vi "Add cell to tableV2.vi"(0 "PdfP Table":refnum<k24>, 1 "Row format with ref":T8, 2 "Image to Add [ ]":T9, 3 "Back Ground Color":u32(colorbox)=16777215, 5 "String [ ]":string[](array[string]), 7 "i":i32, 9 "Column Width (points)":dbl, 11 "error in (no error)":errorcluster, 13 "PDF Report IN":refnum<class "PDF Report Class.lvclass">) -> (4 "PdfP Table duplicate":refnum<k24>, 15 "error out":errorcluster)   [LabVIEW 2019]
doc: "Version 1.0\nDeveloped by Jean-Marc Simard\nCopyright © 2010, Exaprom Inc.\nAll rights reserved.\nLicense: BSD\n\nWith iTextSharp 4.1.6 (http://itextsharp.sourceforge.net)\nunder Mozilla Public License Version 1.1\n(http://www.mozilla.org/MPL/MPL-1.1.html)"
uses:
  C:/work/niobrara_lv/labview pdf writer fixing/DLL/itextsharp.dll
  DLL/itextsharp.dll
  Controls/Font Controls/Font size.ctl
  Controls/Table Controls/Cell Vertical alignment.ctl
  Controls/Text Controls/Texte alignement.ctl
  Controls/General Controls/Image to Add refnum [ ].ctl
  Controls/Table Controls/Table Custom type Titles or Datas.ctl
  Controls/Text Controls/Unicode/Character type.ctl
  Controls/Text Controls/Unicode/Writing direction.ctl
  Controls/Text Controls/Unicode/ASCII or Unicode.ctl
  LV Class/PDF Report Class/PDF Report Class.lvclass
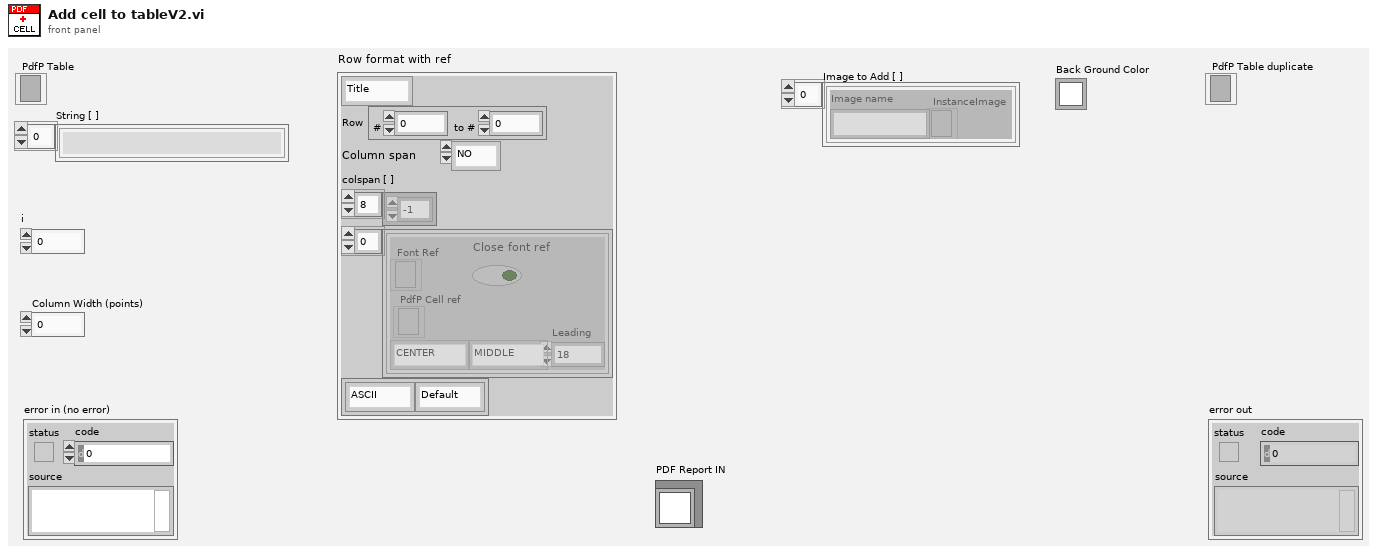
[diagram p1: front panel]
types:
  T1 = typedef "Table Custom type Titles or Datas.ctl" = enum16{"Title", "Data"}
  T2 = typedef "Font size.ctl" = sgl
  T3 = typedef "Texte alignement.ctl" = enum16{"Select", "CENTER", "JUSTIFY", "LEFT", "RIGHT"}
  T4 = typedef "Cell Vertical alignment.ctl" = enum16{"TOP", "MIDDLE", "BOTTOM"}
  T5 = typedef "ASCII or Unicode.ctl" = cluster{"Type":T6, "Direction":T7}
  T6 = typedef "Character type.ctl" = enum16{"ASCII", "Unicode"}
  T7 = typedef "Writing direction.ctl" = enum16{"Default", "NO BIDI", "LTR", "RTL"}
  T8 = cluster{"Titles or datas":T1, "Row":cluster{"#":i16, "to #":i16}, "Column span":enum16{"NO", "YES"}, "colspan [ ]":i8[], "Cell [ ]":cluster{"Font Ref":refnum<k24>, "Leading":T2, "PdfP Cell ref":refnum<k24>, "Horizontal":T3, "Vertical":T4, "Close font ref":bool}[], "ASCII or Unicode":T5}
  T9 = typedef "Image to Add refnum [ ].ctl" = cluster{"Image name":string, "InstanceImage":refnum<k24>}[]
  T10 = cluster{"Font Ref":refnum<k24>, "Leading":T2, "PdfP Cell ref":refnum<k24>, "Horizontal":T3, "Vertical":T4, "Close font ref":bool}[]
  T11 = cluster{"Font Ref":refnum<k24>, "Leading":T2, "PdfP Cell ref":refnum<k24>, "Horizontal":T3, "Vertical":T4, "Close font ref":bool}
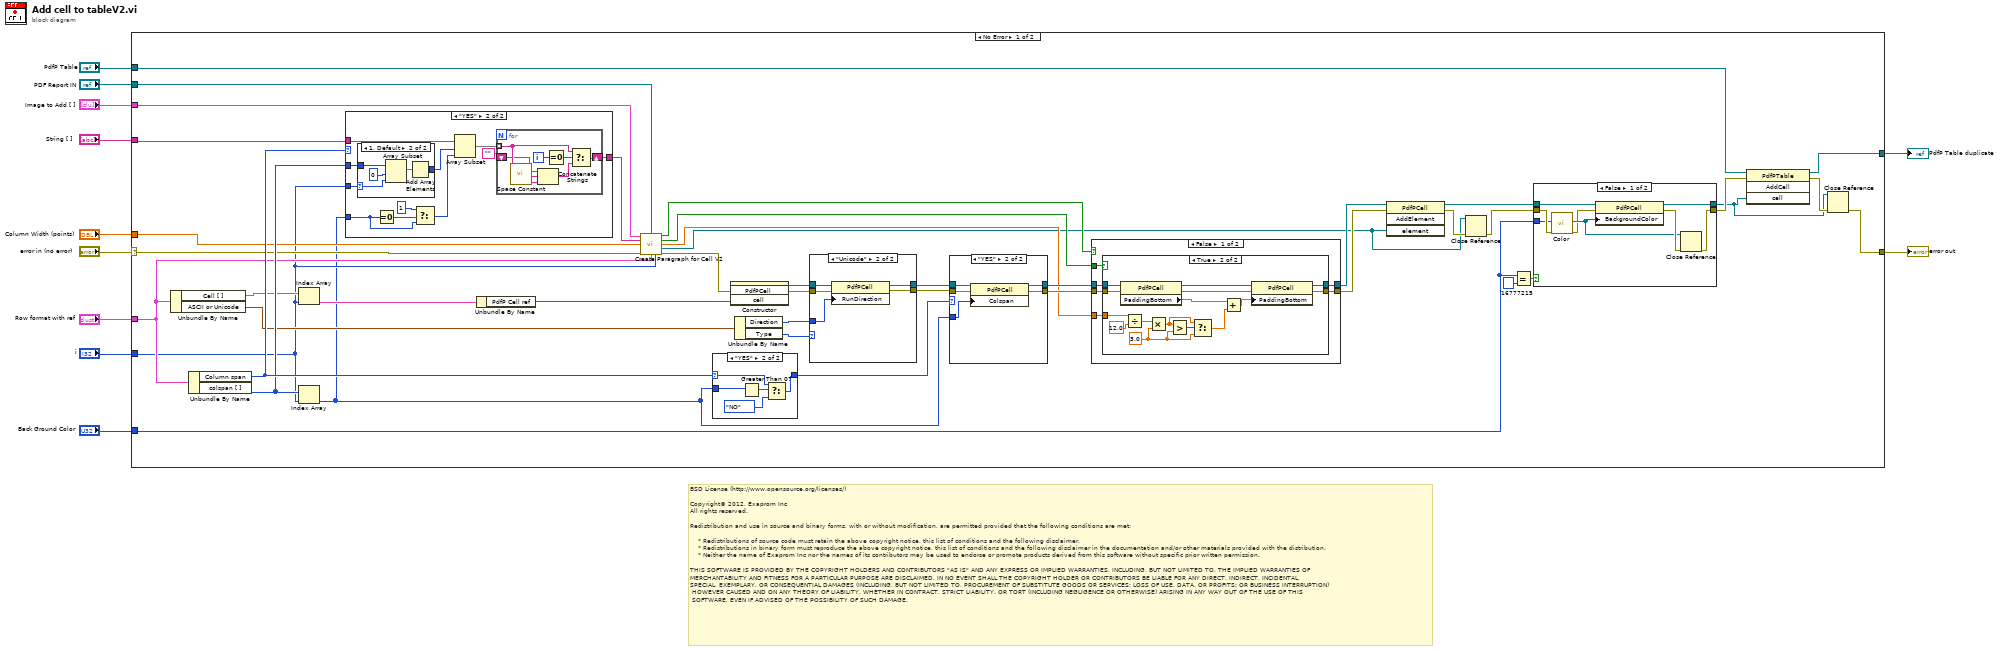
[diagram p0: block diagram]
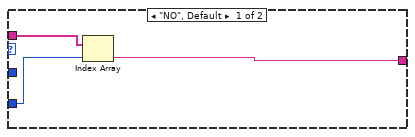
[diagram p2: hidden frame]
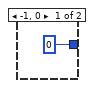
[diagram p3: hidden frame]
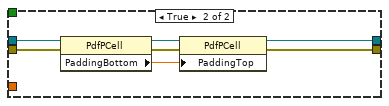
[diagram p8: hidden frame]
diagram:
  # "BSD License (http://www.opensource.org/licenses/)\n\nCopyright© 2012, Exaprom Inc\nAll rights reserved.\n\nRedistribution and use in source and binary forms, with or without modification, are permitted provided that the following conditions are met:\n\n    * Redistributions of source code must retain the above copyright notice, this list of conditions and the following disclaimer.\n    * Redistributions in binary form must reproduce the above copyright notice, this list of conditions and the following disclaimer in the documentation and/or other materials provided with the distribution.\n    * Neither the name of Exaprom Inc nor the names of its contributors may be used to endorse or promote products derived from this software without specific prior written permission.\n\nTHIS SOFTWARE IS PROVIDED BY THE COPYRIGHT HOLDERS AND CONTRIBUTORS \"AS IS\" AND ANY EXPRESS OR IMPLIED WARRANTIES, INCLUDING, BUT NOT LIMITED TO, THE IMPLIED WARRANTIES OF \nMERCHANTABILITY AND FITNESS FOR A PARTICULAR PURPOSE ARE DISCLAIMED. IN NO EVENT SHALL THE COPYRIGHT HOLDER OR CONTRIBUTORS BE LIABLE FOR ANY DIRECT, INDIRECT, INCIDENTAL,\nSPECIAL, EXEMPLARY, OR CONSEQUENTIAL DAMAGES (INCLUDING, BUT NOT LIMITED TO, PROCUREMENT OF SUBSTITUTE GOODS OR SERVICES; LOSS OF USE, DATA, OR PROFITS; OR BUSINESS INTERRUPTION)\n HOWEVER CAUSED AND ON ANY THEORY OF LIABILITY, WHETHER IN CONTRACT, STRICT LIABILITY, OR TORT (INCLUDING NEGLIGENCE OR OTHERWISE) ARISING IN ANY WAY OUT OF THE USE OF THIS\n SOFTWARE, EVEN IF ADVISED OF THE POSSIBILITY OF SUCH DAMAGE."
  n1 = case shown="No Error" "error in (no error)" {
    selector: "error in (no error)" -> [w20 w143]
    tunnel: [w45 w143] -> w10
    tunnel: [w52 w142] -> w9
    tunnel: "PdfP Table" -> [w27 w142]
    tunnel: "String [ ]" -> [w16 _]
    tunnel: "Image to Add [ ]" -> [w18 _]
    tunnel: "Column Width (points)" -> [w19 _]
    tunnel: "i" -> [w15 _]
    tunnel: "Back Ground Color" -> [w41 _]
    tunnel: "Row format with ref" -> [w17 _]
    tunnel: "PDF Report IN" -> [w12 _]
    frame No Error {
      n2 = Unbundle By Name(w17) -> ("Cell [ ]"=w39:T10, "ASCII or Unicode"=w21:T5)
      n3 = Unbundle By Name(w17) -> ("Column span"=w54:enum16{"NO", "YES"}, "colspan [ ]"=w53:i8[])
      n4 = Index Array(array=w39, index=w15) -> (element=w30:T11)
      n5 = Index Array(array=w53, index=w15) -> (element=w14:i8)
      n6 = case shown="\"YES\"" w54 {
        tunnel: w53 -> [_ w68]
        tunnel: [w55 w58] -> w13
        tunnel: w16 -> [w56 w66]
        tunnel: w15 -> [w57 w65]
        tunnel: w14 -> [_ w61]
        frame "NO", Default {
          n7 = Index Array(array=w56, index=w57) -> (element=w55:string)
        }
        frame "YES" {
          n8 = case shown="1, Default" w65 {
            selector: w65 -> [_ w77]
            tunnel: w68 -> [_ w81]
            tunnel: [i8 0 ("span") w78] -> w67
            frame -1, 0 {
            }
            frame 1, Default {
              n9 = Array Subset(array=w81, index=0, length=w77) -> (w79:i8[])
              n10 = Add Array Elements(numeric array=w79) -> (sum=w78:i8)
            }
          }
          n11 = Equal To 0?(x=w61) -> (x = 0?=w64:bool)
          n12 = Select(t=i8 1, s=w64, f=w61) -> (s? t:f=w62:i8)
          n13 = Array Subset(array=w66, index=w67, length=w62) -> (w59:string[])
          n14 = for {
            tunnel: w59 -> [w72] mode=indexing
            shift-right: [w74] -> w58
            shift-left: "" -> [w71]
            i -> [w75]
            n15 = call <vilib>:"Space Constant.vi"() -> ("String"=w70:string)
            n16 = Concatenate Strings(w71, w70, w72) -> (w69:string)
            n17 = Equal To 0?(x=w75) -> (x = 0?=w73:bool)
            n18 = Select(t=w72, s=w73, f=w69) -> (s? t:f=w74:string)
          }
        }
      }
      n19 = Unbundle By Name(w30) -> ("PdfP Cell ref"=w38:refnum<k24>)
      n20 = call <vilib>:"Create Paragraph for Cell V2.vi"("Image to Add [ ]"=w18, "PDF Report IN"=w12, "String"=w13, "Column Width (points)"=w19, "error in (no error)"=w20, "Row format with ref"=w17, "i"=w15) -> ("Valid Image?"=w24:bool, "Modify Padding?"=w25:bool, "Font Size"=w26:sgl, "Paragraph refnum"=w22:refnum<k24>, "error out"=w23:errorcluster)  [unwired: 4 in]
      n21 = case shown="\"YES\"" w54 {
        selector: w54 -> [w96 w99]
        tunnel: w14 -> [_ w101]
        tunnel: [w96 w97] -> w35
        frame "NO", Default {
        }
        frame "YES" {
          n22 = Greater Than 0?(x=w101) -> (x > 0?=w100:bool)
          n23 = Select(t=w99, s=w100, f=enum16{"NO", "YES"}."NO") -> (s? t:f=w97:enum16{"NO", "YES"})
        }
      }
      n24 = constructor class="PdfPCell"(error in=w23, "cell"=w38) -> (reference out=w34:refnum<k24>, error out=w33:errorcluster)  [unwired: 2 in, 2 out]
      n25 = Unbundle By Name(w21) -> ("Direction"=w28:T7, "Type"=w29:T6)
      n26 = case shown="\"Unicode\"" w29 {
        tunnel: w34 -> [w83 w88]
        tunnel: w33 -> [w82 w87]
        tunnel: [w82 w86] -> w32
        tunnel: [w83 w85] -> w31
        tunnel: w28 -> [_ w84]
        frame "ASCII", Default {
        }
        frame "Unicode" {
          n27 = property class="PdfPCell"(reference=w88, error in=w87, "RunDirection"=w84) -> (reference out=w85:refnum<k24>, error out=w86:errorcluster)
        }
      }
      n28 = case shown="\"YES\"" w35 {
        tunnel: w31 -> [w90 w95]
        tunnel: w32 -> [w89 w94]
        tunnel: [w90 w93] -> w37
        tunnel: [w89 w92] -> w36
        tunnel: w14 -> [_ w91]
        frame "NO", Default {
        }
        frame "YES" {
          n29 = property class="PdfPCell"(reference=w95, error in=w94, "Colspan"=w91) -> (reference out=w93:refnum<k24>, error out=w92:errorcluster)
        }
      }
      n30 = case shown="False" w24 {
        tunnel: w36 -> [w104 w129]
        tunnel: [w103 w128] -> w43
        tunnel: w37 -> [w105 w127]
        tunnel: [w106 w125] -> w42
        tunnel: w25 -> [w107 _]
        tunnel: w26 -> [w102 _]
        frame False {
          n31 = case shown="True" w107 {
            tunnel: [w109 w122] -> w106
            tunnel: w105 -> [w109 w120]
            tunnel: w104 -> [w108 w119]
            tunnel: [w108 w121] -> w103
            tunnel: w102 -> [_ w116]
            frame False {
            }
            frame True {
              w111 = sgl 3.0 ("y")
              n32 = property class="PdfPCell"(reference=w120, error in=w119) -> (reference out=w123:refnum<k24>, error out=w124:errorcluster, "PaddingBottom"=w118:sgl)
              n33 = Divide(x=w116, y=sgl 12.0) -> (x/y=w114:sgl)
              n34 = Multiply(x=w114, y=w111) -> (x*y=w112:sgl)
              n35 = Greater?(x=w112, y=w111) -> (0:w113:bool)
              n36 = Select(t=w112, s=w113, f=w111) -> (s? t:f=w110:sgl)
              n37 = Add(x=w118, y=w110) -> (x+y=w117:sgl)
              n38 = property class="PdfPCell"(reference=w123, error in=w124, "PaddingBottom"=w117) -> (reference out=w122:refnum<k24>, error out=w121:errorcluster)
            }
          }
        }
        frame True {
          n39 = property class="PdfPCell"(reference=w127, error in=w129) -> (reference out=w126:refnum<k24>, error out=w130:errorcluster, "PaddingBottom"=w131:sgl)
          n40 = property class="PdfPCell"(reference=w126, error in=w130, "PaddingTop"=w131) -> (reference out=w125:refnum<k24>, error out=w128:errorcluster)
        }
      }
      n41 = invoke class="PdfPCell" method="AddElement"(reference=w42, error in=w43, "element"=w22) -> (reference out=w40:refnum<k24>, error out=w48:errorcluster)  [unwired: 1 in, 2 out]
      n42 = Close Reference(reference=w22, error in (no error)=w48) -> (error out=w47:errorcluster)
      n43 = Equal?(x=w41, y=u32 16777215 ("Color")) -> (x = y?=w50:bool)
      n44 = case shown="False" w50 {
        tunnel: w40 -> [w139 w141]
        tunnel: w47 -> [w134 w140]
        tunnel: [w138 w141] -> w44
        tunnel: [w136 w140] -> w49
        tunnel: w41 -> [w133 _]
        frame False {
          n45 = call "Color.vi"("error in (no error)"=w134, "Color"=w133) -> ("error out"=w132:errorcluster, "Color"=w135:refnum<k24>)  [unwired: 8 out]
          n46 = property class="PdfPCell"(reference=w139, error in=w132, "BackgroundColor"=w135) -> (reference out=w138:refnum<k24>, error out=w137:errorcluster)
          n47 = Close Reference(reference=w135, error in (no error)=w137) -> (error out=w136:errorcluster)
        }
        frame True {
        }
      }
      n48 = invoke class="PdfPTable" method="AddCell"(reference=w27, error in=w49, "cell"=w44) -> (reference out=w52:refnum<k24>, error out=w46:errorcluster)  [unwired: 1 in, 2 out]
      n49 = Close Reference(reference=w44, error in (no error)=w46) -> (error out=w45:errorcluster)
    }
    frame Error {
    }
  }
  "error out" <- w10
  "PdfP Table duplicate" <- w9
